vi "sub_solve3x3submatrix.vi"(10 "solver (in)":cluster{"solved":bool, "values":string[]}[][](array[cluster]) caption="solver array", 11 "puzzle (in)":string[][](array[string])=[["", "1", "", "", "", "", "", ""], ["", "", "6", "", "", "", "6", ""], ["", "", "", "", "6", "", "", ""], ["", "", "", "", "", "", "", ""], ["2", "", "", "6", "7", "", "", "9"], ["", "6", "", "", "", "", "", ""], ["", "6", "", "", "4", "", "", ""], ["", "", "", "", "", "", "", ""], ["", "3", "", "", "2", "", "", "3"]]) -> (2 "solver (out)":cluster{"solved":bool, "values":string[]}[][](array[cluster]))   [LabVIEW 2018]
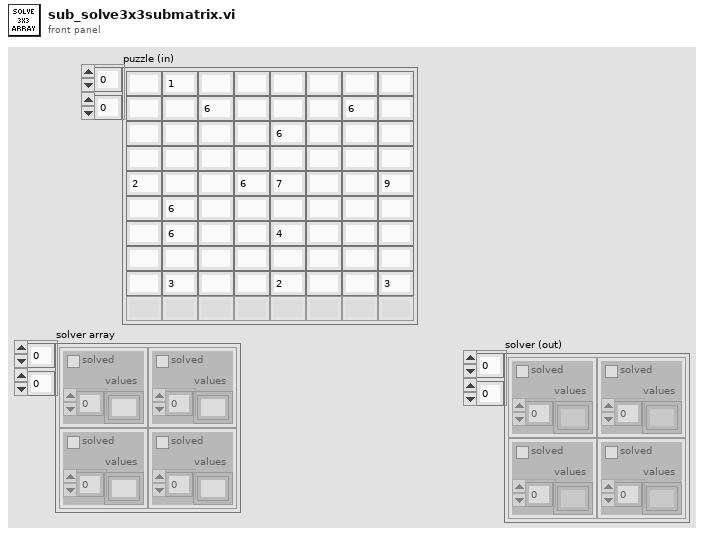
[diagram p1: front panel]
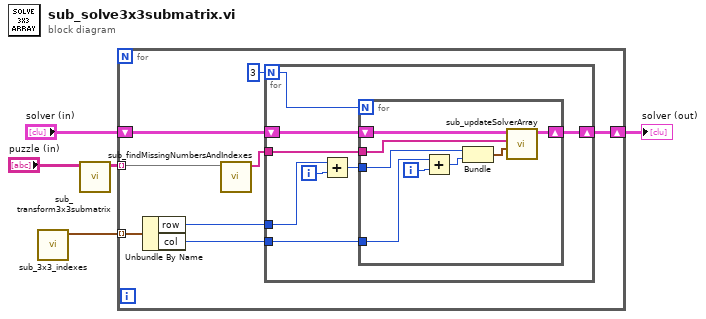
[diagram p0: block diagram]
diagram:
  n1 = call "sub_3x3_indexes.vi"() -> ("3x3 matrix indexes"=w3:cluster{"row":i32, "col":i32}[])  [unwired: 11 in]
  n2 = call "sub_transform3x3submatrix.vi"("puzzle (in)"="puzzle (in)") -> ("transformed submatrix"=w1:string[][])  [unwired: 10 in]
  n3 = for {
    tunnel: w3 -> [w9] mode=indexing
    shift-right: [w8] -> w5
    shift-left: "solver (in)" -> [w7]
    tunnel: w1 -> [w6] mode=indexing
    n4 = Unbundle By Name(w9) -> ("row"=w12:i32, "col"=w11:i32)
    n5 = call "sub_findMissingNumbersAndIndexes.vi"("row (in)"=w6) -> ("missing numbers"=w10:string[])  [unwired: 9 in, 1 out]
    n6 = for {
      N: 3 -> [w20]
      tunnel: w11 -> [w21]
      tunnel: w12 -> [w19]
      shift-right: [w15] -> w8
      shift-left: w7 -> [w16]
      tunnel: w10 -> [w14]
      i -> [w18]
      n7 = Add(x=w19, y=w18) -> (x+y=w17:i32)
      n8 = for {
        N: w20 -> [_]
        tunnel: w21 -> [w28]
        tunnel: w17 -> [w26]
        shift-right: [w23] -> w15
        shift-left: w16 -> [w24]
        tunnel: w14 -> [w22]
        i -> [w29]
        n9 = Add(x=w28, y=w29) -> (x+y=w27:i32)
        n10 = Bundle(w26, w27) -> (w25:cluster{i32, i32})  [unwired: 1 in]
        n11 = call "sub_updateSolverArray.vi"("array index"=w25, "possible candidates"=w22, "solver (in)"=w24) -> ("solver (out)"=w23:cluster{"solved":bool, "values":string[]}[][])  [unwired: 8 in]
      }
    }
  }
  "solver (out)" <- w5
